vi "CreatefolderandTDMS.vi"(0 "object in":refnum<class "Experiment2.lvclass">, 2 "Experiment Series":path, 5 "error in (no error)":errorcluster) -> (14 "object out":refnum<class "Experiment2.lvclass">, 19 "error out":errorcluster)   [LabVIEW 2021, in "Experiment2.lvclass"]
uses:
  Experiment2.lvclass
  Experiment2.lvclass/Experiment2.ctl
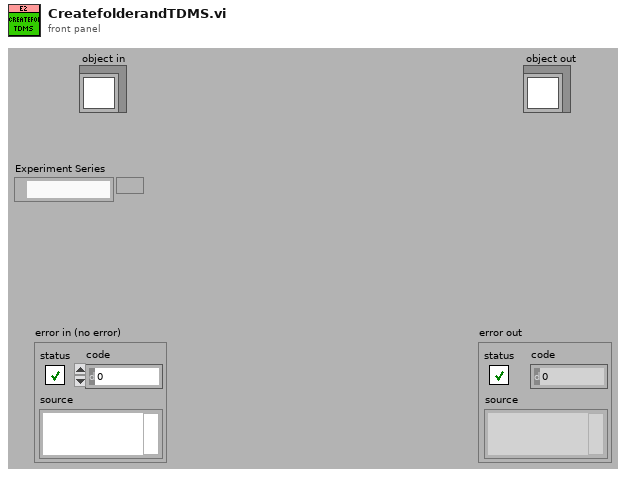
[diagram p1: front panel]
types:
  T1 = enum16{"open", "open or create", "create or replace", "create", "open (read-only)"}
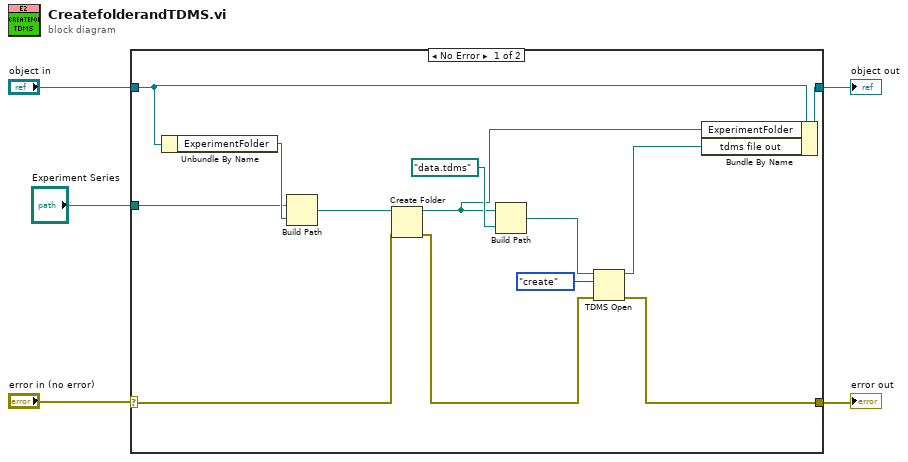
[diagram p0: block diagram]
diagram:
  n1 = case shown="No Error" "error in (no error)" {
    selector: "error in (no error)" -> [w13 w19]
    tunnel: "object in" -> [w17 w20]
    tunnel: [w18 w20] -> w4
    tunnel: [w8 w19] -> w2
    tunnel: "Experiment Series" -> [w15 _]
    frame No Error {
      n2 = Unbundle By Name(w17) -> ("ExperimentFolder"=w16:path)
      n3 = Build Path(base path=w15, name or relative path=w16) -> (appended path=w14:path)
      n4 = Create Folder(path (use dialog)=w14, error in=w13) -> (created path=w6:path, error out=w9:errorcluster)  [unwired: 1 in, 1 out]
      n5 = Build Path(base path=w6, name or relative path=path "data.tdms") -> (appended path=w10:path)
      n6 = TDMS Open(8:w9, 10:T1."create" ("operation (0:open)"), 11:w10) -> (0:w8:errorcluster, 3:w7:refnum<k34>)  [unwired: 4 in]
      n7 = Bundle By Name(cluster=w17, "ExperimentFolder"=w6, "tdms file out"=w7) -> (w18:refnum<class "Experiment2.lvclass">)
    }
    frame Error {
    }
  }
  "object out" <- w4
  "error out" <- w2
